vi "LV86_Get Dimensions.vi"(3 "Image In":T1 {"Dialogs" format="%.0b"}) -> (0 "Dimensions":cluster{"Width":i32, "Height":i32}, 1 "Image Out":T1 {"Dialogs" format="%.0b"})   [LabVIEW 2024]
doc: "This VI gets the dimensions of an image"
uses:
  <userlib>/ImageProcessing/QTLIB_2595_LV86/QT_Image.ctl
panel:
  # "This VI gets the dimensions of an image"
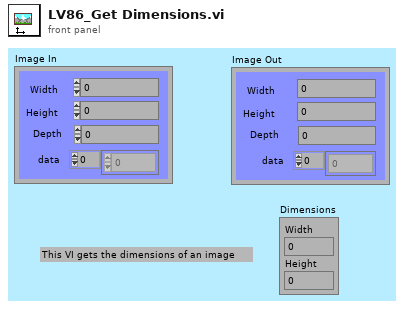
[diagram p1: front panel]
types:
  T1 = typedef "QT_Image.ctl" = cluster{"Width":i32, "Height":i32, "Depth":i32, "data":u8[], "Compressed data":u8[], "Color table":u32[], "Duration":i32, "Options":i32, "Timestamp":i32, "ID":i32, "Reserved":i32, "Dialogs":u32}
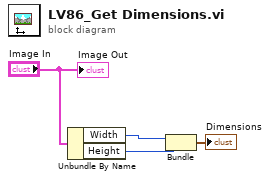
[diagram p0: block diagram]
diagram:
  n1 = Unbundle By Name("Image In") -> ("Width"=w3:i32, "Height"=w2:i32)
  n2 = Bundle("Width"=w3, "Height"=w2) -> (→"Dimensions":cluster{"Width":i32, "Height":i32})  [unwired: 1 in]
  "Image Out" <- "Image In"
